vi "visit.vi"(0 "HGF_Visitor":refnum<class "HGF_Visitor.lvclass">, 2 "HGF_Visitable":refnum<class "HGF_Visitable.lvclass">, 5 "error in (no error)":errorcluster) -> (14 "dup HGF_Visitor":refnum<class "HGF_Visitor.lvclass">, 16 "dup HGF_Visitable":refnum<class "HGF_Visitable.lvclass">, 19 "error out":errorcluster)   [LabVIEW 2014, in "HGF_BaseClasses.lvlib" / "HGF_Visitor.lvclass"]
doc: "This is a static VI that is called from Visitable.accept(). It will call Visitor.action() to perform the requested action which means: calling public methods of Visitable child class."
uses:
  HGF_Visitor.lvclass
  HGF_Visitable/HGF_Visitable.lvclass
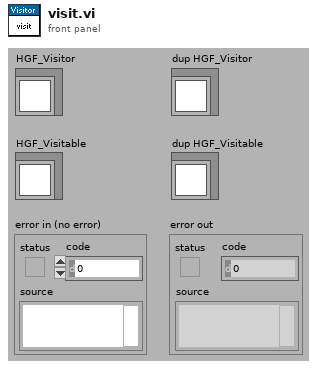
[diagram p1: front panel]
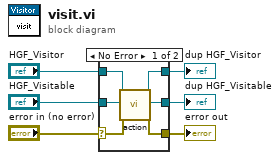
[diagram p0: block diagram]
diagram:
  n1 = case shown="No Error" "error in (no error)" {
    selector: "error in (no error)" -> [w7 w15]
    tunnel: [w10 w15] -> w5
    tunnel: [w12 w14] -> w3
    tunnel: "HGF_Visitor" -> [w8 w14]
    tunnel: [w11 w13] -> w2
    tunnel: "HGF_Visitable" -> [w9 w13]
    frame No Error {
      n2 = call-dynamic "action.vi"("HGF_Visitor in"=w8, "HGF_Visitable"=w9, "error in (no error)"=w7) -> ("HGF_Visitor out"=w12:refnum<class "HGF_Visitor.lvclass">, "dup HGF_Visitable"=w11:refnum<class "HGF_Visitable.lvclass">, "error out"=w10:errorcluster)  [unwired: 14 out]
    }
    frame Error {
    }
  }
  "error out" <- w5
  "dup HGF_Visitor" <- w3
  "dup HGF_Visitable" <- w2
